vi "set_up_graph_hardware_window_properties.vi"(9 "Graph Properties":T1, 11 "Hardware Window Refnum":refnum<vi>) -> ()   [LabVIEW 2020, in "3DPC_SurfacePlot.xctl"]
uses:
  <vilib>/Native 3D Graph/xcontrol/3DPC_SurfacePlot.xctl
  <vilib>/Native 3D Graph/typedefs/prop_graph.ctl
  <vilib>/picture/3D Picture Control/NI_3D Picture Control.lvlib
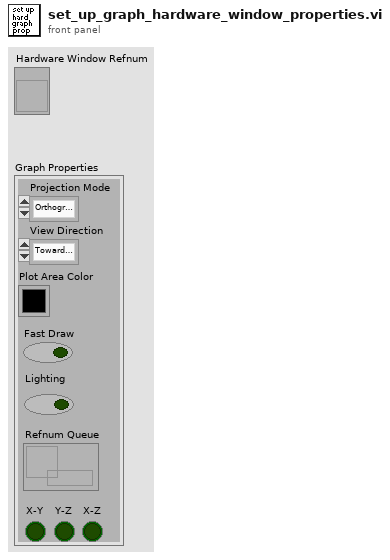
[diagram p1: front panel]
types:
  T1 = typedef "3DPC_SurfacePlot.xctl/prop_graph.ctl" = cluster{"Projection Mode":enum16{"Orthographic", "Perspective"}, "View Direction":enum32{"Towards X-Y Plane", "Towards Y-Z Plane", "Towards X-Z Plane", "User Define"}, "Plot Area Color":u32, "Fast Draw":bool, "X-Y":bool, "Y-Z":bool, "X-Z":bool, "Lighting":bool, "Refnum Queue":refnum<queue>}
  T2 = enum32{"Towards X-Y Plane", "Towards Y-Z Plane", "Towards X-Z Plane", "User Define"}
  T3 = enum16{"None", "Spherical", "Flying", "Oriented"}
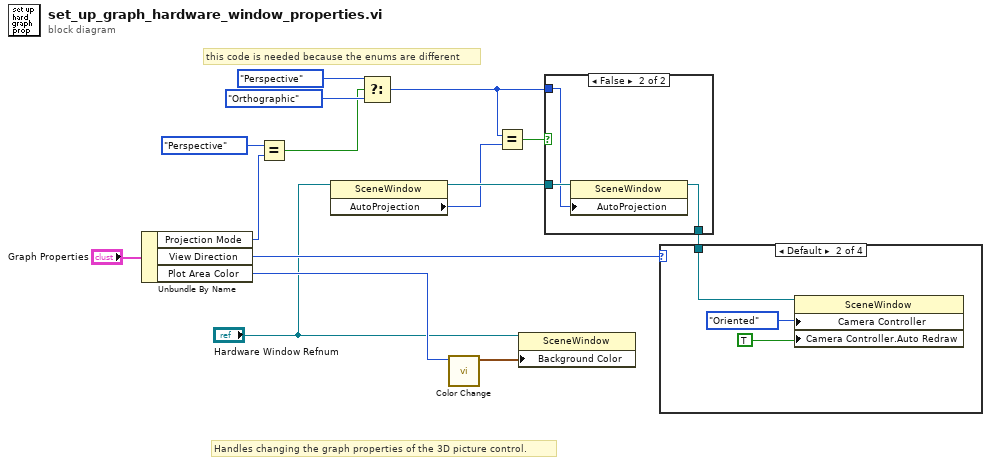
[diagram p0: block diagram]
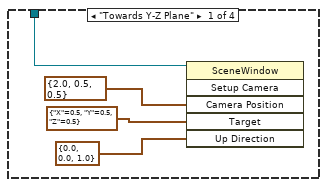
[diagram p2: hidden frame]
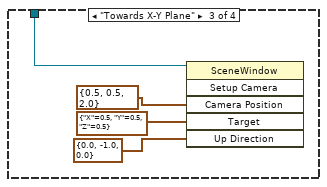
[diagram p3: hidden frame]
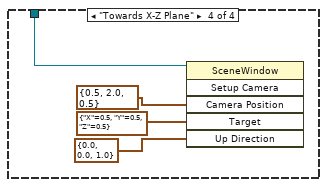
[diagram p4: hidden frame]
diagram:
  # "this code is needed because the enums are different"
  # "Handles changing the graph properties of the 3D picture control."
  n1 = Unbundle By Name("Graph Properties") -> ("Projection Mode"=w6:enum16{"Orthographic", "Perspective"}, "View Direction"=w14:T2, "Plot Area Color"=w13:u32)
  n2 = Equal?(x=enum16{"Orthographic", "Perspective"}."Perspective", y=w6) -> (x = y?=w4:bool)
  n3 = property class="SceneWindow"(reference="Hardware Window Refnum") -> (reference out=w10:refnum<vi>, "AutoProjection"=w2:enum16{"None", "Perspective", "Orthographic"})  [unwired: 1 in, 1 out]
  n4 = Select(t=enum16{"None", "Perspective", "Orthographic"}."Perspective" ("Automatic Projection Mode"), s=w4, f=enum16{"None", "Perspective", "Orthographic"}."Orthographic" ("Automatic Projection Mode")) -> (s? t:f=w1:enum16{"None", "Perspective", "Orthographic"})
  n5 = call <vilib>:"Color Change.vi"("Color"=w13) -> ("RGBA"=w12:cluster{"R":sgl, "G":sgl, "B":sgl, "A":sgl})  [unwired: 1 in, 9 out]
  n6 = Equal?(x=w1, y=w2) -> (x = y?=w11:bool)
  n7 = property on="Property Node" class="SceneWindow"(reference="Hardware Window Refnum", "Background Color"=w12) -> ()  [unwired: 1 in, 2 out]
  n8 = case shown="False" w11 {
    tunnel: [w16 w17] -> w9
    tunnel: w10 -> [w16 w19]
    tunnel: w1 -> [_ w18]
    frame True {
    }
    frame False {
      n9 = property class="SceneWindow"(reference=w19, "AutoProjection"=w18) -> (reference out=w17:refnum<vi>)  [unwired: 1 in, 1 out]
    }
  }
  n10 = case shown="Default" w14 {
    tunnel: w9 -> [w20 w25 w27 w31]
    frame "Towards Y-Z Plane" {
      n11 = invoke class="SceneWindow" method="Setup Camera"(reference=w20, "Camera Position"=cluster{"X":sgl, "Y":sgl, "Z":sgl} {"X"=2.0, "Y"=0.5, "Z"=0.5}, "Target"=cluster{"X":sgl, "Y":sgl, "Z":sgl} {"X"=0.5, "Y"=0.5, "Z"=0.5} ("Camera Position"), "Up Direction"=cluster{"X":sgl, "Y":sgl, "Z":sgl} {"X"=0.0, "Y"=0.0, "Z"=1.0} ("Camera Position")) -> ()  [unwired: 2 in, 6 out]
    }
    frame Default {
      n12 = property class="SceneWindow"(reference=w25, "Camera Controller"=T3."Oriented" ("Camera Controller:Type"), "Camera Controller.Auto Redraw"=TRUE ("Camera Controller:Auto Redraw")) -> ()  [unwired: 1 in, 2 out]
    }
    frame "Towards X-Y Plane" {
      n13 = invoke class="SceneWindow" method="Setup Camera"(reference=w27, "Camera Position"=cluster{"X":sgl, "Y":sgl, "Z":sgl} {"X"=0.5, "Y"=0.5, "Z"=2.0}, "Target"=cluster{"X":sgl, "Y":sgl, "Z":sgl} {"X"=0.5, "Y"=0.5, "Z"=0.5} ("Camera Position"), "Up Direction"=cluster{"X":sgl, "Y":sgl, "Z":sgl} {"X"=0.0, "Y"=-1.0, "Z"=0.0} ("Camera Position")) -> ()  [unwired: 2 in, 6 out]
    }
    frame "Towards X-Z Plane" {
      n14 = invoke class="SceneWindow" method="Setup Camera"(reference=w31, "Camera Position"=cluster{"X":sgl, "Y":sgl, "Z":sgl} {"X"=0.5, "Y"=2.0, "Z"=0.5}, "Target"=cluster{"X":sgl, "Y":sgl, "Z":sgl} {"X"=0.5, "Y"=0.5, "Z"=0.5} ("Camera Position"), "Up Direction"=cluster{"X":sgl, "Y":sgl, "Z":sgl} {"X"=0.0, "Y"=0.0, "Z"=1.0} ("Camera Position")) -> ()  [unwired: 2 in, 6 out]
    }
  }
